vi "Load Data.vi"(8 "error in (no error)":errorcluster, 11 "Data Directory":path=path "C:/Users/LAV-UFSC-2023/Documents/LAV-TCC/Dados-Experimentos/Dados-Bancada-LABVIEW") -> (0 "error out":errorcluster, 3 "New Graph Data":waveform(dbl)[](array[waveform]))   [LabVIEW 2022 SP3]
doc: "Loads data from a file on disk."
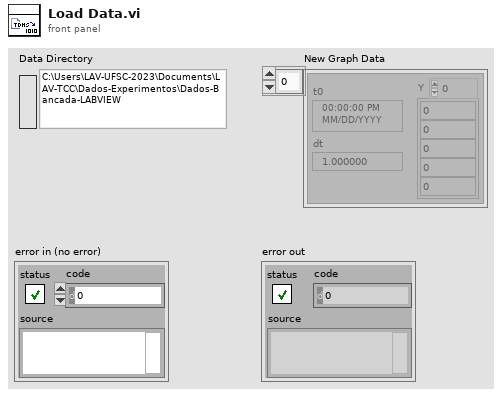
[diagram p1: front panel]
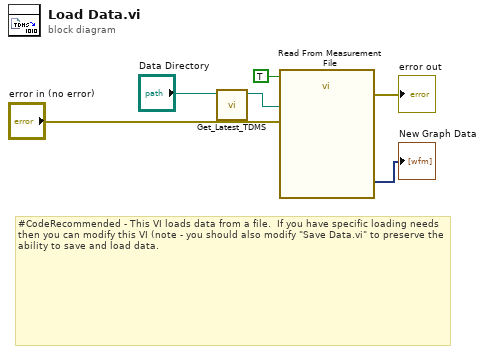
[diagram p0: block diagram]
diagram:
  # "#CodeRecommended - This VI loads data from a file.  If you have specific loading needs then you can modify this VI (note - you should also modify \"Save Data.vi\" to preserve the ability to save and load data."
  n1 = call "Get_Latest_TDMS.vi"("Data Directory"="Data Directory") -> ("Latest_TDMS_File_Path"=w3:path)  [unwired: 10 in]
  n2 = call "Read From Measurement File"("error in (no error)"="error in (no error)", "Filename"=w3, "Reset"=TRUE) -> ("error out"=→"error out":errorcluster, "Signals"=→"New Graph Data":dynamicdata)  [unwired: 3 in, 4 out]
